vi "校准页面.vi"() -> ()   [LabVIEW 2016, in "斯坦道多参数.lvlib"]
panel:
  in  "信号值":dbl
  in  "多列列表框":i32(listbox)
  in  "标准值":dbl caption="标液一："
  in  "校准方式":u16(ring) caption="校准方式：" items=["单点校准", "两点校准", "三点校准"]
  in  "校准参数":u16(ring) caption="校准参数：" items=["水温", "pH", "溶解氧"]
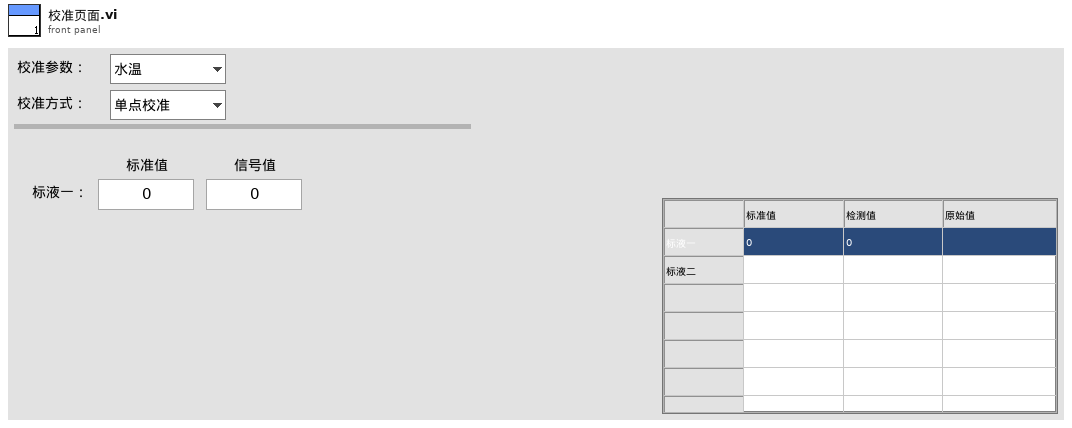
[diagram p1: front panel]
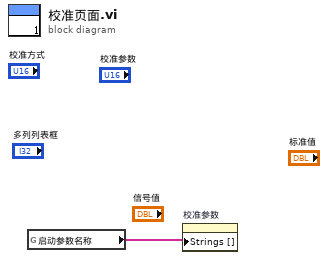
[diagram p0: block diagram]
diagram:
  n1 = global read "多参数全局变量.vi" "启动参数名称"() -> (w1:string[])
  n2 = property on="校准参数" class="Ring (严格)"("Strings []"=w1) -> ()  [unwired: 2 in, 2 out]
